vi "Rest_posture_deco.vi"(8 "error in (no error)":errorcluster) -> (0 "error out":errorcluster)   [LabVIEW 2017]
uses:
  3f13d254-2f8f-4e62-b687-dd237a566472.vi
  IP Address.vi
  <vilib>/httpClient/LabVIEWHTTPClient.lvlib
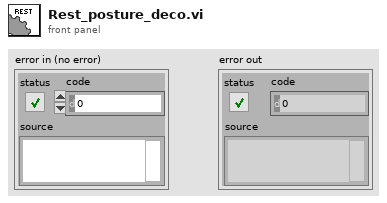
[diagram p1: front panel]
types:
  T1 = enum16{"off", "red", "green", "yellow", "blue", "pink", "cyan", "white"}
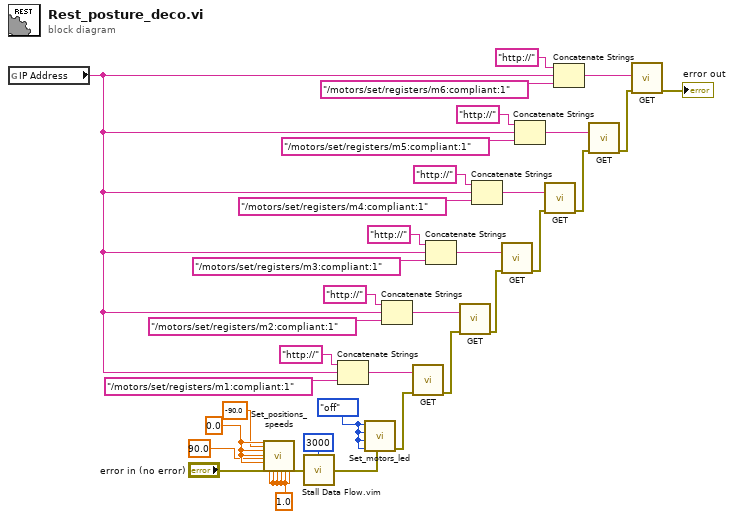
[diagram p0: block diagram]
diagram:
  w26 = 0.0 ("m1")
  w30 = T1."off" ("Color m2")
  w29 = 1.0 ("Speed m5")
  n1 = global read "IP Address.vi" "IP Address"() -> (w1:string)
  n2 = call "Set_positions_speeds.vi"("m1"=w26, "m2"=-90.0, "m3"=w26, "m4"=w26, "m5"=90.0, "m6"=w26, "error in (no error)"="error in (no error)", "Speed m1"=w29, "Speed m2"=w29, "Speed m3"=w29, "Speed m4"=w29, "Speed m5"=w29, "Speed m6"=w29) -> ("error out"=w22:errorcluster)  [unwired: 14 in]
  n3 = call "Stall Data Flow.vim"("value in"=w22, "milliseconds to wait"=u32 3000) -> ("value out"=w21:errorcluster)  [unwired: 1 out]
  n4 = Concatenate Strings("http://" ("string"), w1, "/motors/set/registers/m1:compliant:1" ("string")) -> (w3:string)
  n5 = call "Set_motors_led.vi"("error in (no error)"=w21, "Color m6"=w30, "Color m5"=w30, "Color m3"=w30, "Color m2"=w30) -> ("error out"=w27:errorcluster)  [unwired: 6 in]
  n6 = Concatenate Strings("http://" ("string"), w1, "/motors/set/registers/m2:compliant:1" ("string")) -> (w4:string)
  n7 = call <vilib>:"GET.vi"("url"=w3, "error in (no error)"=w27) -> ("error out"=w31:errorcluster)  [unwired: 10 in, 3 out]
  n8 = Concatenate Strings("http://" ("string"), w1, "/motors/set/registers/m3:compliant:1" ("string")) -> (w5:string)
  n9 = call <vilib>:"GET.vi"("url"=w4, "error in (no error)"=w31) -> ("error out"=w32:errorcluster)  [unwired: 10 in, 3 out]
  n10 = Concatenate Strings("http://" ("string"), w1, "/motors/set/registers/m4:compliant:1" ("string")) -> (w6:string)
  n11 = call <vilib>:"GET.vi"("url"=w5, "error in (no error)"=w32) -> ("error out"=w33:errorcluster)  [unwired: 10 in, 3 out]
  n12 = Concatenate Strings("http://" ("string"), w1, "/motors/set/registers/m5:compliant:1" ("string")) -> (w7:string)
  n13 = call <vilib>:"GET.vi"("url"=w6, "error in (no error)"=w33) -> ("error out"=w34:errorcluster)  [unwired: 10 in, 3 out]
  n14 = Concatenate Strings("http://" ("string"), w1, "/motors/set/registers/m6:compliant:1" ("string")) -> (w8:string)
  n15 = call <vilib>:"GET.vi"("url"=w7, "error in (no error)"=w34) -> ("error out"=w35:errorcluster)  [unwired: 10 in, 3 out]
  n16 = call <vilib>:"GET.vi"("url"=w8, "error in (no error)"=w35) -> ("error out"=→"error out":errorcluster)  [unwired: 10 in, 3 out]
